vi "ROI entry-Get selected Z-plane index.vi"(8 "error in (no error)":errorcluster, 11 "Initialisation":bool) -> (0 "error out":errorcluster, 3 "Z-plane selector (index)":i32)   [LabVIEW 2020]
uses:
  ROI Entry screen/Globals/gl_ROI Entry UI globals.vi
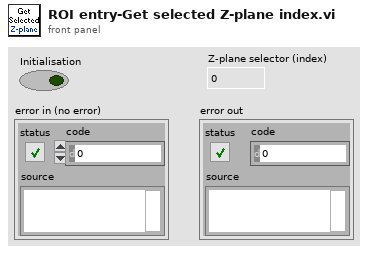
[diagram p1: front panel]
types:
  T1 = typedef "ROI entry screen ctrl refs cluster.ctl" = cluster{"Done button":refnum<vi>, "Imaging button":refnum<vi>, "Acquisition button":refnum<vi>, "Scan dwell time per pixel (us)":refnum<vi>, "# of planes":refnum<vi>, "Zoom Ctrl":refnum<vi>, "Equal size":refnum<vi>, "Channel":refnum<vi>, "Image Display":refnum<vi>, "Z-Plane Selector":refnum<vi>, "Number of lines left":refnum<vi>, "Z-stack folder path":refnum<vi>, "POI Density":refnum<vi>, "Arb Plane Entry":refnum<vi>, "Whole Plane":refnum<vi>, "Line Mode":refnum<vi>, "Clear Last":refnum<vi>, "Clear All":refnum<vi>, "Delete Lines":refnum<vi>, "Trial Length (sec)":refnum<vi>, "Palette Type":refnum<vi>, "Intensity slider":refnum<vi>, "# POI":refnum<vi>, "Max Z Proj":refnum<vi>, "Zplane ind":refnum<vi>, "Wavelength (nm)":refnum<vi>, "Number of Trials":refnum<vi>, "Funct stim.trig.enable":refnum<vi>, "Funct stim.trig.delay (s)":refnum<vi>, "Line Mode":refnum<vi>, "Step size (µm)":refnum<vi>, "ROI move mode":refnum<vi>, "Cool-down time (s)":refnum<vi>, "Enable cool-down time":refnum<vi>, "Motor Z ind. (um)":refnum<vi>, "AOL Z ind. (um)":refnum<vi>, "Load Reference Image":refnum<vi>, "Rel.  Res.":refnum<vi>, "ROI LIST":refnum<vi>, "Show All":refnum<vi>, "ROI Type":refnum<vi>, "Start Plane":refnum<vi>, "Stop Plane":refnum<vi>, "Offset ROI":refnum<vi>, "Tab Control":refnum<vi>, "Laser Power(%)":refnum<vi>, "Cycle rate":refnum<vi>, "FOV (Ind.)":refnum<vi>, "Frame Size (Ind.)":refnum<vi>, "Resolution (Ind.)":refnum<vi>, "Pixel Density (Ind)":refnum<vi>, "Laser Power (Ind.)":refnum<vi>, "Dwell Time (Ind.)":refnum<vi>, "Adj MC":refnum<vi>}
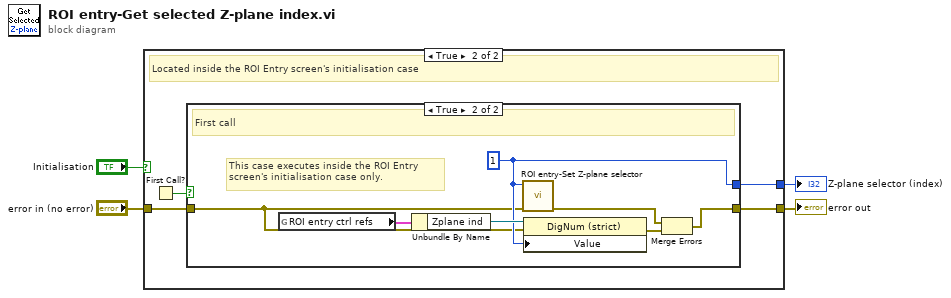
[diagram p0: block diagram]
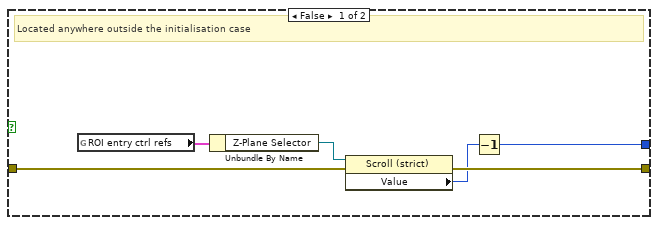
[diagram p2: hidden frame]
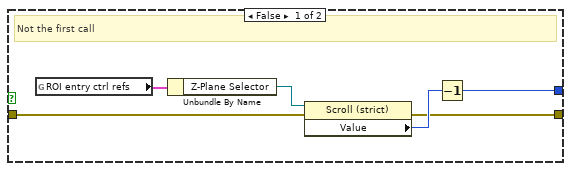
[diagram p3: hidden frame]
diagram:
  n1 = case shown="True" "Initialisation" {
    tunnel: [w8 w12] -> w4
    tunnel: [w6 w13] -> w3
    tunnel: "error in (no error)" -> [w5 w11]
    frame False {
      # "Located anywhere outside the initialisation case"
      n2 = global read "gl_ROI Entry UI globals.vi" "ROI entry ctrl refs"() -> (w9:T1)
      n3 = Unbundle By Name(w9) -> ("Z-Plane Selector"=w10:refnum<vi>)
      n4 = property on="Property Node" class="Scroll (strict)"(reference=w10, error in=w5) -> (error out=w8:errorcluster, "Value"=w7:i32)  [unwired: 1 out]
      n5 = Decrement(x=w7) -> (x-1=w6:i32)
    }
    frame True {
      # "Located inside the ROI Entry screen's initialisation case"
      n6 = First Call?() -> (First Call?: T/F=w14:bool)
      n7 = case shown="True" w14 {
        tunnel: [w16 w25] -> w13
        tunnel: [w17 w21] -> w12
        tunnel: w11 -> [w15 w24]
        frame False {
          # "Not the first call"
          n8 = global read "gl_ROI Entry UI globals.vi" "ROI entry ctrl refs"() -> (w19:T1)
          n9 = Unbundle By Name(w19) -> ("Z-Plane Selector"=w20:refnum<vi>)
          n10 = property on="Property Node" class="Scroll (strict)"(reference=w20, error in=w15) -> (error out=w17:errorcluster, "Value"=w18:i32)  [unwired: 1 out]
          n11 = Decrement(x=w18) -> (x-1=w16:i32)
        }
        frame True {
          w25 = 1 ("Z-Plane Selector")
          # "This case executes inside the ROI Entry screen's initialisation case only."
          # "First call"
          n12 = global read "gl_ROI Entry UI globals.vi" "ROI entry ctrl refs"() -> (w26:T1)
          n13 = Unbundle By Name(w26) -> ("Zplane ind"=w27:refnum<vi>)
          n14 = call "ROI entry-Set Z-plane selector.vi"("error in (no error)"=w24, "Z-plane selector value"=w25) -> ("error out"=w22:errorcluster)  [unwired: 9 in]
          n15 = property on="Property Node" class="DigNum (strict)"(reference=w27, error in=w24, "Value"=w25) -> (error out=w23:errorcluster)  [unwired: 1 out]
          n16 = Merge Errors(w22, w23) -> (w21:errorcluster)
        }
      }
    }
  }
  "error out" <- w4
  "Z-plane selector (index)" <- w3
